vi "质控参数设置.vi"(11 "质控参数设置":T1) -> (3 "输出簇":T2)   [LabVIEW 2016, in "氨氮.lvlib"]
uses:
  <vilib>/Utility/miscctls.llb/LVPointTypeDef.ctl
panel:
  in  "取消":bool
  in  "确定":bool
  in  "标准液标准浓度":dbl
  in  "跨度标准液浓度":dbl
  in  "零点标准液浓度":dbl
  in  "跨度值":dbl
  # "质控参数设置"
  # "监测参数"
  # "氨氮"
  # "跨度值"
  # "零点核查标准液浓度"
  # "跨度核查标准液浓度"
  # "标样核查标准液浓度"
  # "质控参数设置"
  # "监测参数"
  # "氨氮"
  # "跨度值"
  # "零点核查标准液浓度"
  # "跨度核查标准液浓度"
  # "标样核查标准液浓度"
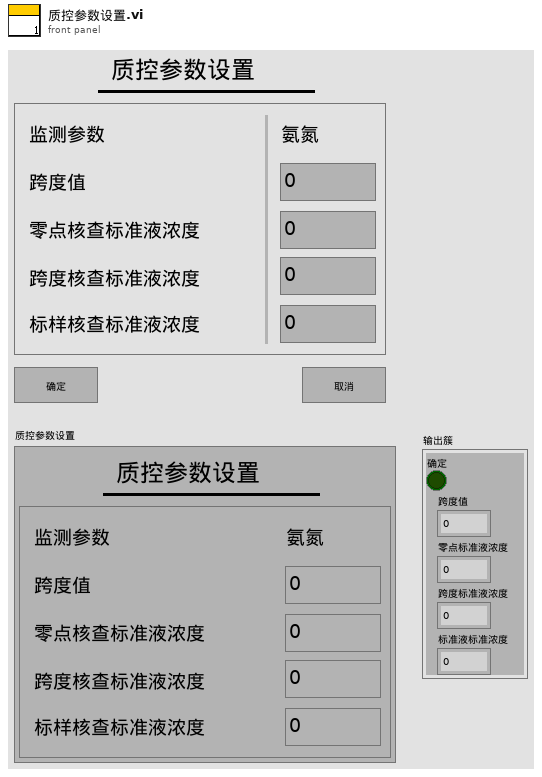
[diagram p1: front panel]
types:
  T1 = cluster{"跨度值":dbl, "零点标准液浓度":dbl, "跨度标准液浓度":dbl, "标准液标准浓度":dbl}
  T2 = cluster{"确定":bool, "跨度值":dbl, "零点标准液浓度":dbl, "跨度标准液浓度":dbl, "标准液标准浓度":dbl}
  T3 = typedef "LVPointTypeDef.ctl" = cluster{"Horizontal":i16, "Vertical":i16}
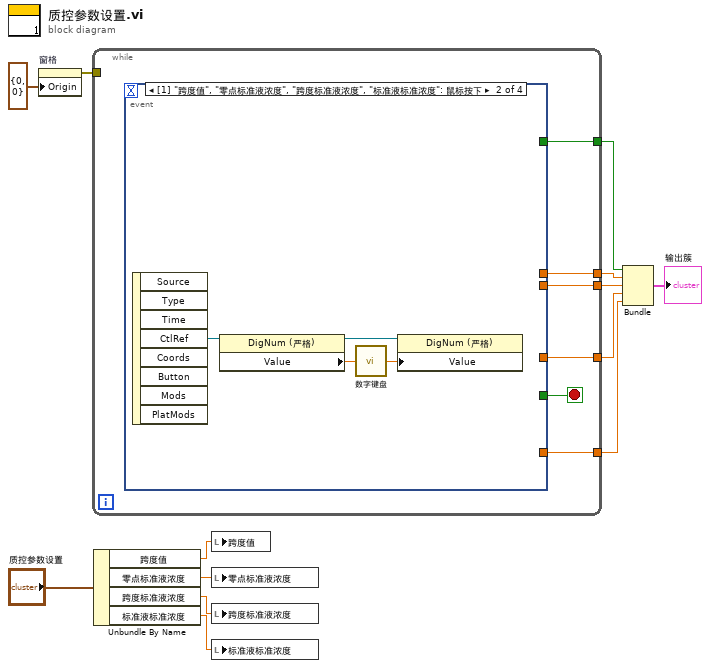
[diagram p0: block diagram]
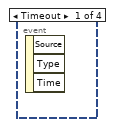
[diagram p2: hidden frame]
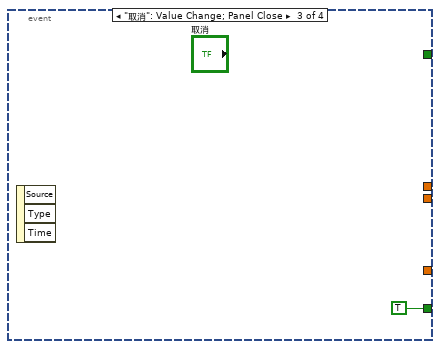
[diagram p3: hidden frame]
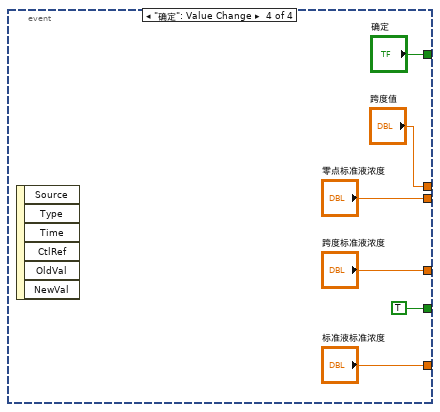
[diagram p4: hidden frame]
diagram:
  n1 = property on="窗格" class="Pane"("Origin"=T3 {"Horizontal"=0, "Vertical"=0} ("原点")) -> (error out=w12:errorcluster)  [unwired: 2 in, 1 out]
  n2 = while {
    tunnel: w12 -> [_]
    tunnel: [w18] -> w11
    tunnel: [w17] -> w10
    tunnel: [w16] -> w9
    tunnel: [w15] -> w8
    tunnel: [w14] -> w7
    stop <- w19 stop-if-true
    n3 = event shown="[1] \"跨度值\", \"零点标准液浓度\", \"跨度标准液浓度\", \"标准液标准浓度\": 鼠标按下" {
      selector: _ -> [_ _ _ _]
      dyn-events: _ -> [_ _ _ _]
      timeout: _ -> [_ _ _ _]
      tunnel: [_ _ TRUE TRUE] -> w19
      tunnel: [_ _ _ "跨度值"] -> w18
      tunnel: [_ _ _ "零点标准液浓度"] -> w17
      tunnel: [_ _ _ "跨度标准液浓度"] -> w16
      tunnel: [_ _ _ "标准液标准浓度"] -> w15
      tunnel: [_ _ _ "确定"] -> w14
      event Timeout {
        n4 = event-data() -> ()  [unwired: 1 in, 3 out]
      }
      event "跨度值", "零点标准液浓度", "跨度标准液浓度", "标准液标准浓度": Mouse Down {
        n5 = event-data() -> ("CtlRef"=w23:refnum<vi>)  [unwired: 1 in, 7 out]
        n6 = property class="DigNum (严格)"(reference=w23) -> (reference out=w21:refnum<vi>, "Value"=w22:dbl)  [unwired: 1 in, 1 out]
        n7 = call "数字键盘.vi"("OldNumber"=w22) -> ("NewNumber"=w20:dbl)
        n8 = property class="DigNum (严格)"(reference=w21, "Value"=w20) -> ()  [unwired: 1 in, 2 out]
      }
      event "取消": Value Change; Panel Close {
        n9 = event-data() -> ()  [unwired: 1 in, 3 out]
      }
      event "确定": Value Change {
        n10 = event-data() -> ()  [unwired: 1 in, 6 out]
      }
    }
  }
  n11 = Unbundle By Name("质控参数设置") -> ("跨度值"=w4:dbl, "零点标准液浓度"=w3:dbl, "跨度标准液浓度"=w2:dbl, "标准液标准浓度"=w1:dbl)
  n12 = local write "跨度值"(w4) -> ()
  n13 = local write "零点标准液浓度"(w3) -> ()
  n14 = local write "跨度标准液浓度"(w2) -> ()
  n15 = local write "标准液标准浓度"(w1) -> ()
  n16 = Bundle("确定"=w7, "跨度值"=w11, "零点标准液浓度"=w10, "跨度标准液浓度"=w9, "标准液标准浓度"=w8) -> (→"输出簇":T2)  [unwired: 1 in]
